vi "Asylum_Driver_SendObjectDataToLithography.vi"(8 "error in (no error)":errorcluster, 10 "Pattern Data":T2, 11 "User Event in":refnum<user-event>) -> (0 "error out":errorcluster)   [LabVIEW 2019]
uses:
  <userlib>/LevyLab/Relay Box/Typedefs/Resistor--enum.ctl
  <userlib>/LevyLab/Relay Box/Relay-Box.lvclass
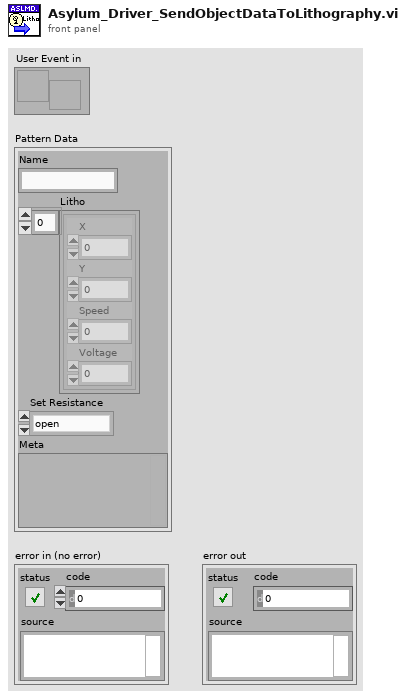
[diagram p1: front panel]
types:
  T1 = typedef "Relay-Box.lvclass/Resistor--enum.ctl" = enum16{"open", "discharge tip", "0 ohms", "100k ohm", "10M ohm", "1G ohm"}
  T2 = cluster{"Name":string, "Litho":cluster{"X":dbl, "Y":dbl, "Speed":dbl, "Voltage":dbl}[], "Set Resistance":T1, "Meta":variant}
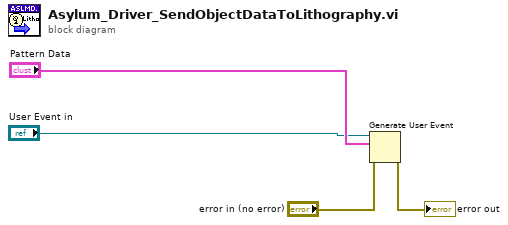
[diagram p0: block diagram]
diagram:
  n1 = Generate User Event(user event="User Event in", event data cluster="Pattern Data", error in="error in (no error)") -> (error out=→"error out":errorcluster)  [unwired: 1 in, 1 out]
